vi "Newtons_Square_Root.vi"() -> ()   [LabVIEW 2022 SP3]
panel:
  out "Number of Iterations":i32
  in  "Percent Difference":dbl=0.001 format="%#_13g"
  out "Calculated Y":dbl
  in  "X":dbl
  # "Newton's Root:\nEnter a value for X. Newton's Iterative method\nfor calculating square roots will be used to produce a value Y = sqrt(X).\nThe number of iterations required to produce a value of Y within the \nentered percent difference will be displayed as well."
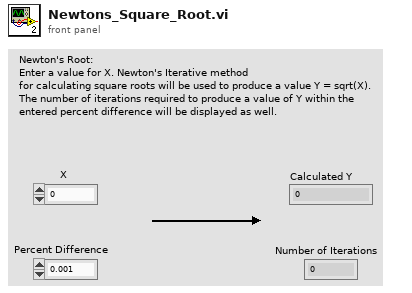
[diagram p1: front panel]
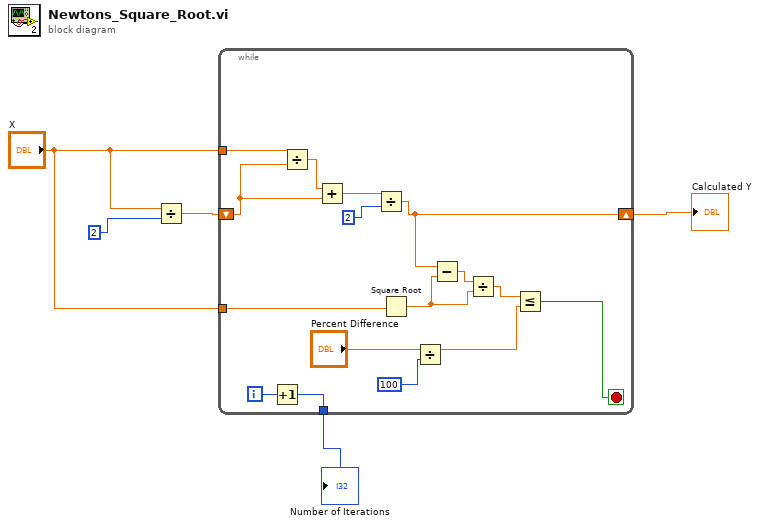
[diagram p0: block diagram]
diagram:
  n1 = Divide(x="X", y=2) -> (x/y=w4:dbl)
  n2 = while {
    shift-right: [w15] -> w2
    shift-left: w4 -> [w19]
    tunnel: "X" -> [w21]
    tunnel: "X" -> [w16]
    tunnel: [w6] -> w1
    i -> [w7]
    stop <- w10 stop-if-true
    n3 = Increment(x=w7) -> (x+1=w6:i32)
    n4 = Divide(x=w21, y=w19) -> (x/y=w20:dbl)
    n5 = Add(x=w20, y=w19) -> (x+y=w18:dbl)
    n6 = Divide(x=w18, y=2) -> (x/y=w15:dbl)
    n7 = Square Root(x=w16) -> (sqrt(x)=w14:dbl)
    n8 = Divide(x="Percent Difference", y=100) -> (x/y=w9:dbl)
    n9 = Subtract(x=w15, y=w14) -> (x-y=w13:dbl)
    n10 = Divide(x=w13, y=w14) -> (x/y=w12:dbl)
    n11 = Less Or Equal?(x=w12, y=w9) -> (x <= y?=w10:bool)
  }
  "Calculated Y" <- w2
  "Number of Iterations" <- w1
